vi "Disconnect.vi"(8 "error in (no error)":errorcluster, 11 "SQLite3LV Connection in":refnum<class "sqlite3.lvclass">) -> (0 "error out":errorcluster)   [LabVIEW 2014, in "SQLite3LV.lvlib" / "sqlite3.lvclass"]
doc: "Disconnect from an active SQLite3LV Connection connection"
uses:
  sqlite3.lvclass
  sqlite3.lvclass/sqlite3.ctl
  SQLite3LV.lvlib
  sqlite3_64.dll
panel:
  out "zSQL":string
  out "ppDb":i64 format="%.0x"
  out "count":i32
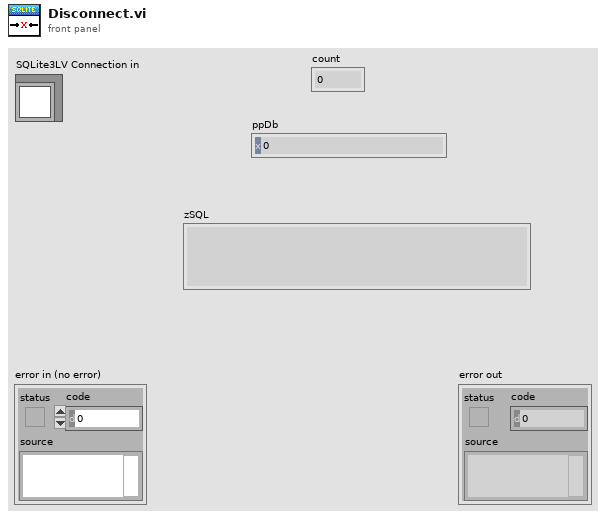
[diagram p1: front panel]
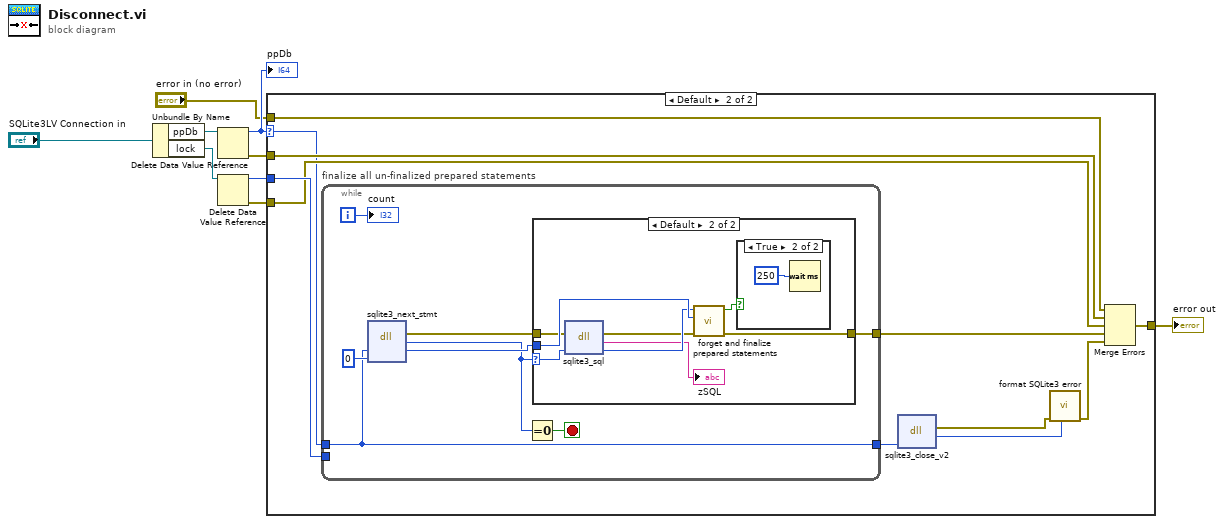
[diagram p0: block diagram]
diagram:
  n1 = Unbundle By Name("SQLite3LV Connection in") -> ("ppDb"=w4:refnum<data-value>, "lock"=w7:refnum<data-value>)
  n2 = Delete Data Value Reference(data value reference=w4) -> (data value=w3:i64, error out=w2:errorcluster)  [unwired: 1 in]
  "ppDb" <- w3
  n3 = Delete Data Value Reference(data value reference=w7) -> (data value=w6:i32, error out=w5:errorcluster)  [unwired: 1 in]
  n4 = case shown="Default" w3 {
    selector: w3 -> [_ w12]
    tunnel: [w10 w21] -> w9
    tunnel: w6 -> [_ w20]
    tunnel: w5 -> [_ w16]
    tunnel: w2 -> [_ w15]
    tunnel: "error in (no error)" -> [w10 w14]
    frame 0 {
    }
    frame Default {
      n5 = while "finalize all un-finalized prepared statements" {
        tunnel: [w29] -> w18
        tunnel: w20 -> [_]
        tunnel: [w25] -> w13
        tunnel: w12 -> [w25]
        i -> [w27]
        stop <- w24 stop-if-true
        n6 = dll-call lib="C:/Users/BobUser/Desktop/LVTables/sqlite3**.*" fn="sqlite3_next_stmt"("ppDb"=w25, "pStmt"=i64 0) -> (error out=w23:errorcluster, "psqlite3_stmt"=w22:i64, "ppDb"=w26:i64)  [unwired: 4 in, 1 out]
        n7 = Equal To 0?(x=w22) -> (x = 0?=w24:bool)
        n8 = case shown="Default" w22 {
          selector: w22 -> [_ w34]
          tunnel: [w30 w38] -> w29
          tunnel: w26 -> [_ w37]
          tunnel: w23 -> [w30 w35]
          frame 0 {
          }
          frame Default {
            n9 = dll-call lib="C:/Users/BobUser/Desktop/LVTables/sqlite3**.*" fn="sqlite3_sql"(error in=w35, "pStmt"=w34) -> (error out=w31:errorcluster, "zSQL"=→"zSQL":string, "pStmt"=w33:i64)  [unwired: 2 in, 1 out]
            n10 = call "forget and finalize prepared statements.vi"("error in (no error)"=w31, "ppDb"=w37, "pStmt"=w33) -> ("error out"=w38:errorcluster, "error?"=w36:bool)  [unwired: 7 in]
            n11 = case shown="True" w36 {
              frame False {
              }
              frame True {
                n12 = Wait (ms)(milliseconds to wait=u32 250) -> ()  [unwired: 1 out]
              }
            }
          }
        }
        "count" <- w27
      }
      n13 = dll-call lib="C:/Users/BobUser/Desktop/LVTables/sqlite3**.*" fn="sqlite3_close_v2"("ppDb"=w13) -> (error out=w17:errorcluster, "return type"=w19:i32)  [unwired: 4 in, 1 out]
      n14 = call "format SQLite3 error.vi"("SQLite3LV Connection result"=w19, "error in (no error)"=w17) -> ("error out"=w11:errorcluster)  [unwired: 9 in]
      n15 = Merge Errors(w14, w15, w16, w18, w11) -> (w21:errorcluster)
    }
  }
  "error out" <- w9
